vi "HXG2_WriteAllCtrl.vi"(6 "All Ctrl Array":dbl[](array[numeric]), 8 "error in":errorcluster, 11 "Analog Task":refnum<k21>) -> (0 "error out":errorcluster)   [LabVIEW 2012]
doc: "This VI passes all values for the control of the system to the write task vi"
uses:
  Modules/EnableAirGly/HXG2enable.ctl
  <vilib>/Analysis/Matrix/Numeric/Conversions/Array To Matrix - RA.vi
  <vilib>/Analysis/baseanly.llb/A x Vector.vi
  <vilib>/DAQmx/write.llb/DAQmx Write (Analog 1D DBL NChan 1Samp).vi
  <vilib>/Analysis/NI_AALBase.lvlib
  <vilib>/Analysis/Matrix/NI_Matrix.lvlib
  <vilib>/DAQmx/write.llb/DAQmx Write (Analog 2D DBL NChan NSamp).vi
panel:
  out "In Range?":bool[](array[boolean])
  out "mA":dbl[](array[numeric])
  out "% Duty Cycle":dbl[](array[numeric])
  out "To Task (mA)":dbl[](array[numeric])
  # "Pre-Dither"
  # "BlowerVFD"
  # "PumpVFD"
  # "BlowerVFD"
  # "ByPass Damper"
  # "PumpVFD"
  # "AirHTR SCR"
  # "ByPass Damper"
  # "EXV Air Evap"
  # "AirHTR SCR"
  # "GlyHTR SCR"
  # "EXV Air Evap"
  # "EXV Gly Evap"
  # "GlyHTR SCR"
  # "EXV Gly Evap"
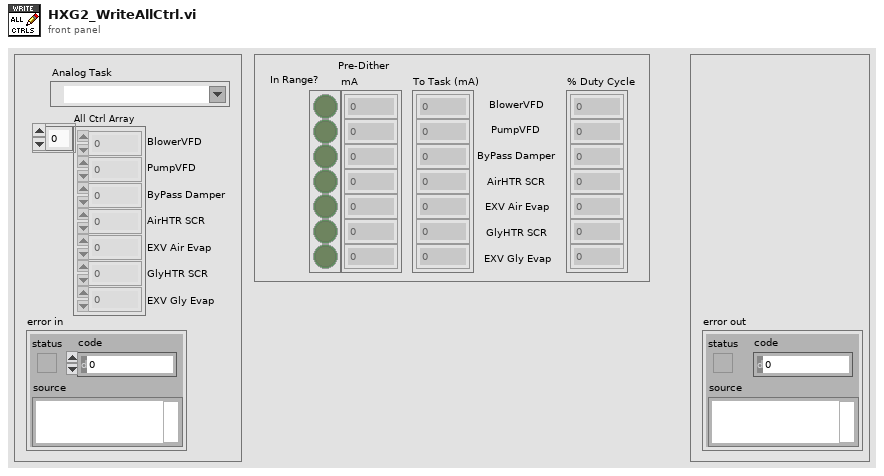
[diagram p1: front panel]
types:
  T1 = typedef "HXG2enable.ctl" = enum16{"Write Refs", "Write", "Pass"}
  T2 = typedef "NI_Matrix.lvlib/RealMatrix.ctl" = dbl[][]
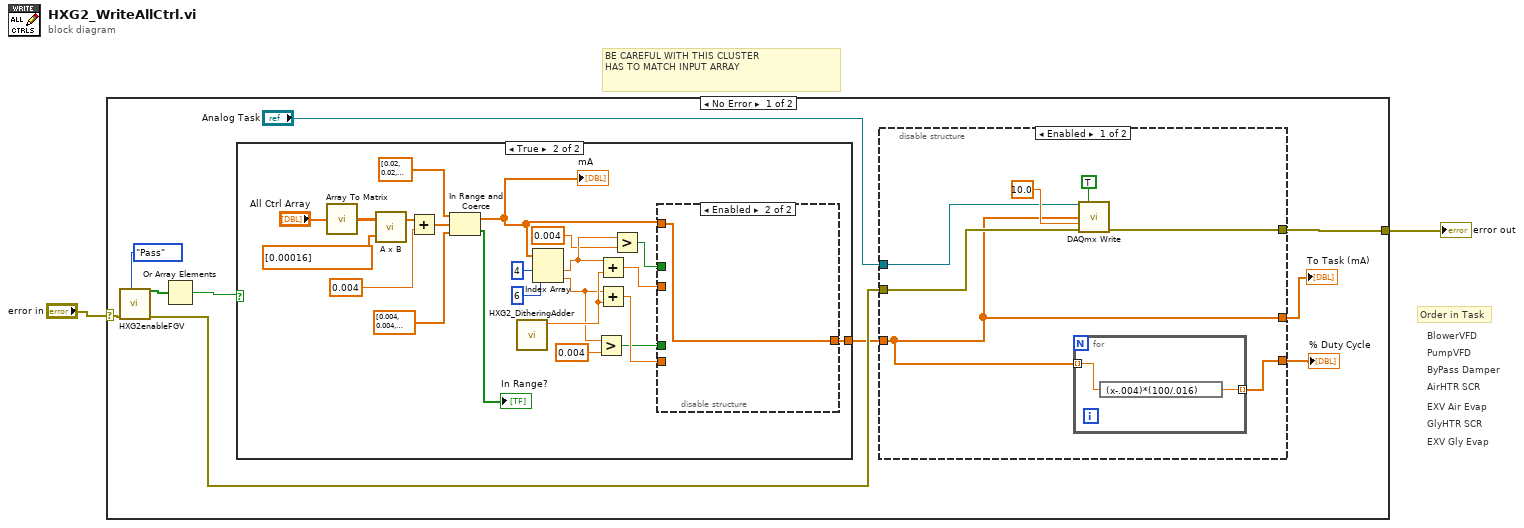
[diagram p0: block diagram]
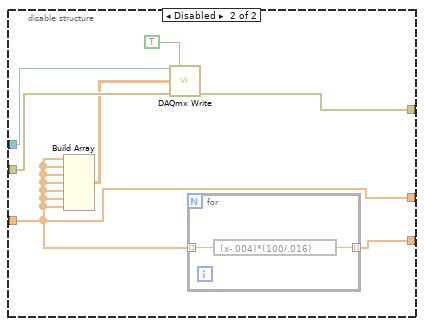
[diagram p2: hidden frame]
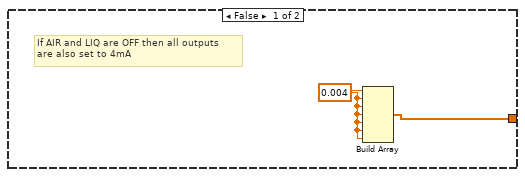
[diagram p3: hidden frame]
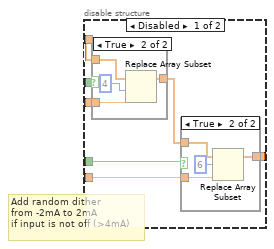
[diagram p4: hidden frame]
diagram:
  # "Order in Task"
  # "EXV Gly Evap"
  # "GlyHTR SCR"
  # "EXV Air Evap"
  # "AirHTR SCR"
  # "ByPass Damper"
  # "PumpVFD"
  # "BlowerVFD"
  # "BE CAREFUL WITH THIS CLUSTER\nHAS TO MATCH INPUT ARRAY"
  n1 = case shown="No Error" "error in" {
    selector: "error in" -> [w9 w73]
    tunnel: [w12 w73] -> w2
    frame No Error {
      n2 = call "HXG2enableFGV.vi"("ENABLE Ctrl"=HXG2enable."Pass", "error in (no error)"=w9) -> ("error out"=w5:errorcluster, "Air-Liq Out"=w8:bool[])  [unwired: 7 in, 1 out]
      n3 = Or Array Elements(Boolean array=w8) -> (logical OR=w7:bool)
      n4 = case shown="True" w7 {
        tunnel: [w31 w43] -> w4
        frame False {
          w32 = 0.004
          # "If AIR and LIQ are OFF then all outputs \nare also set to 4mA"
          n5 = Build Array(w32, w32, w32, w32, w32, w32, w32) -> (w31:dbl[])
        }
        frame True {
          n6 = call-poly <vilib>:"Array To Matrix.vi"("Real 1D Array"="All Ctrl Array") -> ("Real Matrix (Column Vector)"=w53:T2)
          n7 = call-poly <vilib>:"A x B.vi"("Vector"=dbl[] [0.00016] ("V' x A"), "A"=w53) -> ("A x Vector"=w51:dbl[])  [unwired: 1 out]
          n8 = Add(x=w51, y=0.004) -> (x+y=w37:dbl[])
          n9 = In Range and Coerce(upper limit=dbl[] [0.02, 0.02, 0.02, 0.02, 0.02, 0.02, 0.02], x=w37, lower limit=dbl[] [0.004, 0.004, 0.004, 0.004, 0.004, 0.004, 0.004] ("upper limit")) -> (coerced(x)=w36:dbl[], In Range?=→"In Range?":bool[])
          "mA" <- w36
          n10 = call "HXG2_DitheringAdder.vi"() -> ("-.2 to .2 (mA)"=w48:dbl)  [unwired: 11 in]
          n11 = Index Array(array=w36, index #1=4 ("index"), index #2=6 ("index")) -> (element #1=w46:dbl, element #2=w41:dbl)
          n12 = Greater?(x=w41, y=0.004) -> (0:w39:bool)
          n13 = Add(x=w46, y=w48) -> (x+y=w47:dbl)
          n14 = Add(x=w41, y=w48) -> (x+y=w42:dbl)
          n15 = Greater?(x=w46, y=0.004) -> (0:w44:bool)
          n16 = disable-structure shown="Enabled" {
            disable-tunnel: w36 -> [w61 w72]
            disable-tunnel: w47 -> [w60 _]
            disable-tunnel: w44 -> [w59 _]
            disable-tunnel: [w57 w72] -> w43
            disable-tunnel: w42 -> [w56 _]
            disable-tunnel: w39 -> [w55 _]
            frame Disabled {
              # "Add random dither\nfrom -2mA to 2mA\nif input is not off (>4mA)"
              n17 = case shown="True" w59 {
                tunnel: w61 -> [w67 w71]
                tunnel: w60 -> [_ w69]
                tunnel: [w67 w68] -> w58
                frame False {
                }
                frame True {
                  n18 = Replace Array Subset(array=w71, new element=w69, index=4) -> (w68:dbl[])
                }
              }
              n19 = case shown="True" w55 {
                tunnel: w58 -> [w62 w65]
                tunnel: w56 -> [_ w64]
                tunnel: [w62 w63] -> w57
                frame False {
                }
                frame True {
                  n20 = Replace Array Subset(array=w65, new element=w64, index=6) -> (w63:dbl[])
                }
              }
            }
            frame Enabled {
            }
          }
        }
      }
      n21 = disable-structure shown="Enabled" {
        disable-tunnel: [w19 w24] -> w12
        disable-tunnel: [w17 w25] -> w11
        disable-tunnel: "Analog Task" -> [w15 w28]
        disable-tunnel: w5 -> [w14 w26]
        disable-tunnel: w4 -> [w13 w22]
        disable-tunnel: [w13 w22] -> w3
        frame Enabled {
          n22 = for {
            tunnel: [w21] -> w17 mode=indexing
            tunnel: w13 -> [w20] mode=indexing
            n23 = expression code="(x-.004)*(100/.016)"(w20) -> (w21:dbl)
          }
          n24 = call-poly <vilib>:"DAQmx Write.vi"("task/channels in"=w15, "auto start"=TRUE, "data"=w13, "timeout"=10.0, "error in"=w14) -> ("error out"=w19:errorcluster)  [unwired: 8 in, 2 out]
        }
        frame Disabled {
          n25 = Build Array(w22, w22, w22, w22, w22, w22, w22) -> (w23:dbl[][])
          n26 = call-poly <vilib>:"DAQmx Write.vi"("task/channels in"=w28, "auto start"=TRUE, "data"=w23, "error in"=w26) -> ("error out"=w24:errorcluster)  [unwired: 9 in, 2 out]
          n27 = for {
            tunnel: w22 -> [w30] mode=indexing
            tunnel: [w29] -> w25 mode=indexing
            n28 = expression code="(x-.004)*(100/.016)"(w30) -> (w29:dbl)
          }
        }
      }
      "To Task (mA)" <- w3
      "% Duty Cycle" <- w11
    }
    frame Error {
    }
  }
  "error out" <- w2
